vi "OAT Polar Calculate Orbit Coordinats for XY Plot.vi"(6 "polar attributes":T1 {"minimum" format="%.2f"; "maximum" format="%.2f"}, 8 "picture dimensions (w,h)":cluster{"width":i16, "height":i16}, 9 "grid measurements":T2 {"end angle" format="%.2f"; "start angle" format="%.2f"; "scale factors"."b" format="%.2f"; "scale factors"."a" format="%.2f"}, 10 "phases":dbl[](array[numeric]) format="%.2f", 11 "magnitudes":dbl[](array[numeric]) format="%.2f") -> (3 "orbit for XY plot":cluster{"X":dbl[], "Y":dbl[]} {"Y" format="%.2f"; "X" format="%.2f"})   [LabVIEW 2017]
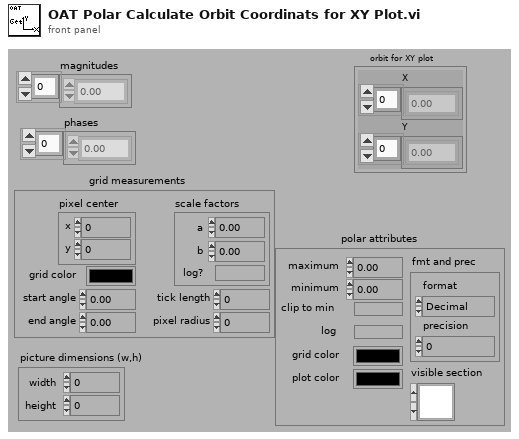
[diagram p1: front panel]
types:
  T1 = cluster{"maximum":dbl, "minimum":dbl, "clip to min":bool, "log":bool, "grid color":u32, "plot color":u32, "fmt and prec":cluster{"format":enum8{"Decimal", "Scientific", "Engineering", "Binary", "Octal", "Hex"}, "precision":u8}, "visible section":u16}
  T2 = cluster{"pixel center":cluster{"x":i16, "y":i16}, "scale factors":cluster{"a":dbl, "b":dbl, "log?":bool}, "grid color":u32, "start angle":dbl, "end angle":dbl, "tick length":i16, "pixel radius":i32}
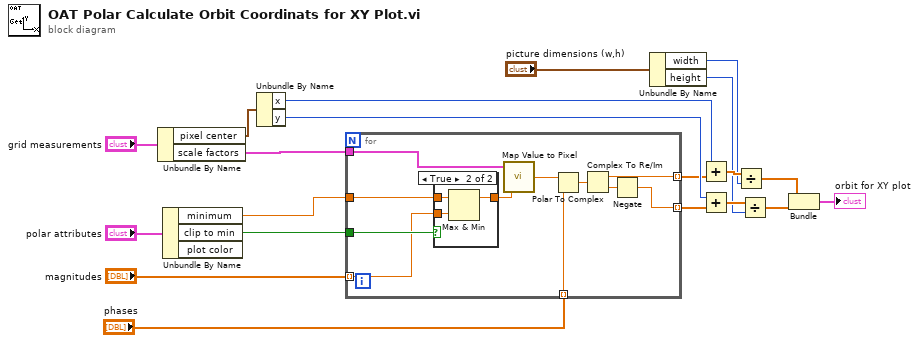
[diagram p0: block diagram]
diagram:
  n1 = Unbundle By Name("grid measurements") -> ("pixel center"=w17:cluster{"x":i16, "y":i16}, "scale factors"=w5:cluster{"a":dbl, "b":dbl, "log?":bool})
  n2 = Unbundle By Name("polar attributes") -> ("minimum"=w18:dbl, "clip to min"=w4:bool)  [unwired: 1 out]
  n3 = Unbundle By Name(w17) -> ("x"=w7:i16, "y"=w16:i16)
  n4 = for {
    tunnel: w18 -> [w31]
    tunnel: "phases" -> [w27] mode=indexing
    tunnel: w5 -> [w26]
    tunnel: w4 -> [w25]
    tunnel: "magnitudes" -> [w24] mode=indexing
    tunnel: [w23] -> w2 mode=indexing
    tunnel: [w22] -> w1 mode=indexing
    n5 = case shown="True" w25 {
      tunnel: w24 -> [w32 w33]
      tunnel: [w32 w34] -> w21
      tunnel: w31 -> [_ w35]
      frame False {
      }
      frame True {
        n6 = Max & Min(x=w35, y=w33) -> (max(x,y)=w34:dbl)  [unwired: 1 out]
      }
    }
    n7 = call <vilib>:"Map Value to Pixel.vi"("x"=w21, "scale factors"=w26) -> ("pixel"=w28:dbl)  [unwired: 1 in]
    n8 = Polar To Complex(1:w27, 2:w28) -> (0:w30:cdb)
    n9 = Complex To Re/Im(x + iy=w30) -> (x=w23:dbl, y=w29:dbl)
    n10 = Negate(x=w29) -> (-x=w22:dbl)
  }
  n11 = Unbundle By Name("picture dimensions (w,h)") -> ("width"=w13:i16, "height"=w11:i16)
  n12 = Add(x=w7, y=w2) -> (x+y=w14:dbl[])
  n13 = Add(x=w16, y=w1) -> (x+y=w12:dbl[])
  n14 = Divide(x=w14, y=w13) -> (x/y=w10:dbl[])
  n15 = Divide(x=w12, y=w11) -> (x/y=w9:dbl[])
  n16 = Bundle(w10, w9) -> (→"orbit for XY plot":cluster{dbl[], dbl[]})  [unwired: 1 in]
